vi "Barrier Wait.vi"(8 "error in (no error)":errorcluster, 11 "Barrier in":T1) -> (0 "error out":errorcluster, 3 "Barrier out":T1)   [LabVIEW 2013, in "POSIX Threads.lvlib" / "Barrier.lvclass"]
uses:
  Barrier.lvclass
  Controls/reference.ctl
  POSIX Thread Object/POSIX Thread Object.lvclass/POSIX Thread Object.ctl
  POSIX Thread Object/Private VIs/libpthread path.vi
  POSIX Thread Object/Private VIs/get pthread error.vi
  POSIX Thread Object/POSIX Thread Object.lvclass
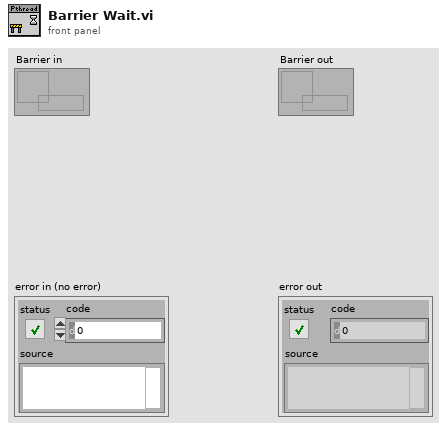
[diagram p1: front panel]
types:
  T1 = typedef "POSIX Threads.lvlib/Barrier.lvclass/reference.ctl" = refnum<data-value>
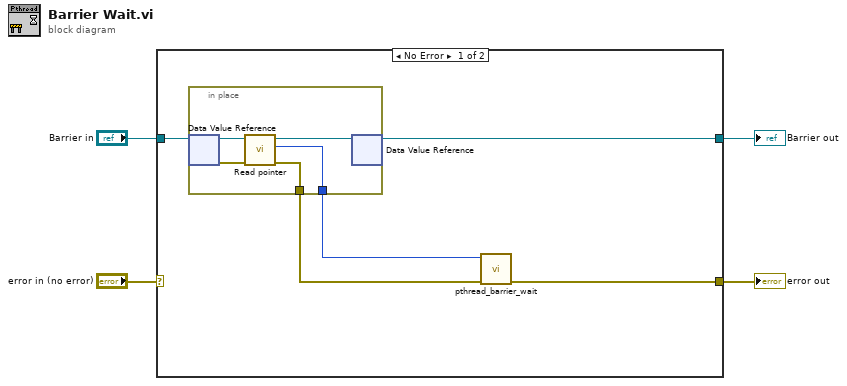
[diagram p0: block diagram]
diagram:
  n1 = case shown="No Error" "error in (no error)" {
    selector: "error in (no error)" -> [_ w16]
    tunnel: [w7 w16] -> w3
    tunnel: "Barrier in" -> [w9 w15]
    tunnel: [w8 w15] -> w1
    frame No Error {
      n2 = in-place {
        in-place-border: [w11] -> w6
        in-place-border: [w10] -> w5
        n3 = in-place-dvr #1(w9) -> (w14:refnum<class "Barrier.lvclass">, w12:errorcluster)
        n4 = call "Read pointer.vi"("error in (no error)"=w12, "POSIX Thread Object in"=w14) -> ("error out"=w11:errorcluster, "pointer"=w10:u64, "POSIX Thread Object out"=w13:refnum<class "Barrier.lvclass">)  [unwired: 7 in]
        n5 = in-place-dvr #1(w13) -> (w8:T1)  [unwired: 1 out]
      }
      n6 = call "pthread_barrier_wait.vi"("error in (no error)"=w6, "barrier ptr in"=w5) -> ("error out"=w7:errorcluster)  [unwired: 8 in, 1 out]
    }
    frame Error {
    }
  }
  "error out" <- w3
  "Barrier out" <- w1
